vi "MiPS_turn_on_heater.vi"(6 "ISOBUS address":T4, 7 "switching_allowed":bool, 8 "error in":errorcluster, 9 "ref_in":T1, 10 "ref_slider":refnum<vi>, 11 "ref_big_msg":refnum<vi>) -> (0 "error out":errorcluster, 3 "ref_out":T1)   [LabVIEW 2019]
uses:
  Mercury iXX Modules/Public/Controls/ISOBus Address.ctl
  Mercury iXX Modules/Public/Controls/Mercury Reference.ctl
  Mercury iXX Modules/Public/Controls/Comms Transport Layer.ctl
  Mercury iXX Modules/Private/Controls/Query Dynamic Reference.ctl
  Mercury iXX Modules/Public/Libraries/Magnet/Controls/Switch Heater.ctl
  Mercury iXX Modules/Public/Libraries/Magnet/Signals/Set/Switch Heater No Check (Set).vi
  Mercury iXX Modules/Public/Libraries/Magnet.lvlib
  Mercury iXX Modules/Mercury iXX.lvlib
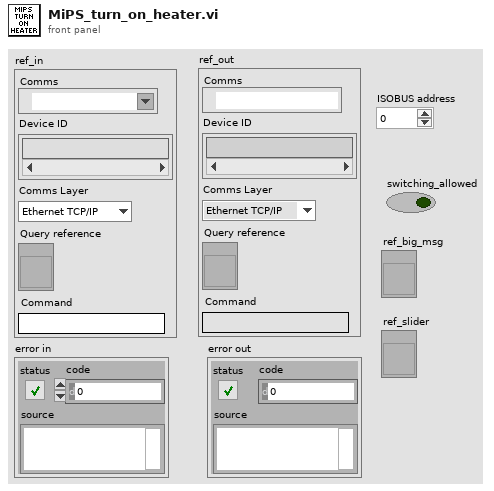
[diagram p1: front panel]
types:
  T1 = typedef "Mercury iXX.lvlib/Mercury Reference.ctl" = cluster{"Comms":refnum<visa-resource-name>, "Device ID":string[], "Comms Layer":T2, "Command":string, "Query reference":T3}
  T2 = typedef "Mercury iXX.lvlib/Comms Transport Layer.ctl" = enum16{"Ethernet TCP/IP", "USB", "ISOBus - RS-232", "GPIB"}
  T3 = typedef "Mercury iXX.lvlib/Query Dynamic Reference.ctl" = refnum<vi>
  T4 = typedef "Mercury iXX.lvlib/ISOBus Address.ctl" = i32
  T5 = typedef "Mercury iXX.lvlib/Magnet.lvlib/Switch Heater.ctl" = string
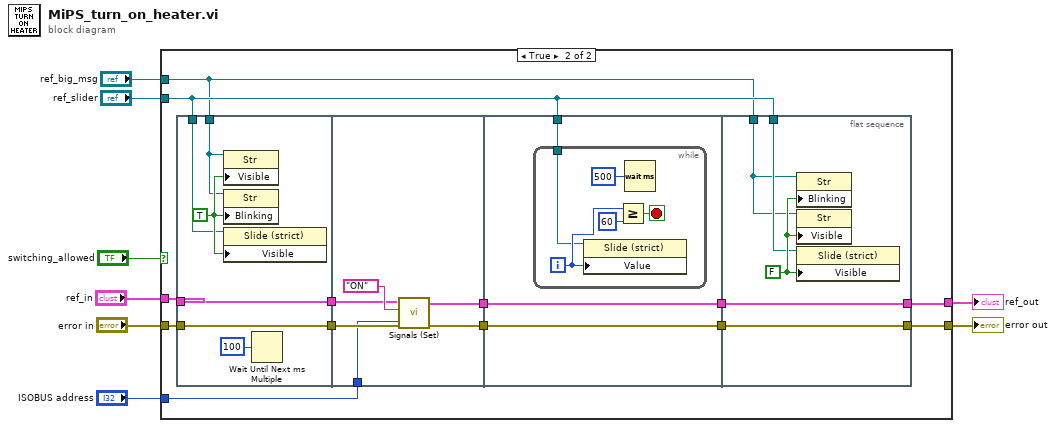
[diagram p0: block diagram]
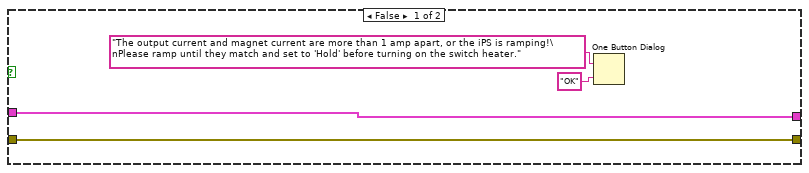
[diagram p2: hidden frame]
diagram:
  n1 = case shown="True" "switching_allowed" {
    tunnel: "ref_in" -> [w12 w20]
    tunnel: [w12 w25] -> w7
    tunnel: "error in" -> [w11 w18]
    tunnel: [w11 w24] -> w6
    tunnel: "ISOBUS address" -> [_ w17]
    tunnel: "ref_slider" -> [_ w14]
    tunnel: "ref_big_msg" -> [_ w13]
    frame False {
      n2 = One Button Dialog(message="The output current and magnet current are more than 1 amp apart, or the iPS is ramping!\nPlease ramp until they match and set to 'Hold' before turning on the switch heater.", button name ("OK")="OK") -> ()  [unwired: 1 out]
    }
    frame True {
      n3 = flat-sequence {
        tunnel: w20 -> [w30]
        tunnel: [w30] -> w21
        tunnel: [w29] -> w19
        tunnel: w18 -> [w29]
        tunnel: w13 -> [w27]
        tunnel: w14 -> [w26]
        tunnel: [w37] -> w16
        tunnel: [w36] -> w15
        tunnel: w21 -> [w34]
        tunnel: w19 -> [w33]
        tunnel: w17 -> [w32]
        tunnel: w16 -> [w40]
        tunnel: w15 -> [w39]
        tunnel: [w40] -> w23
        tunnel: [w39] -> w22
        tunnel: w14 -> [w38]
        tunnel: [w49] -> w24
        tunnel: [w50] -> w25
        tunnel: w23 -> [w50]
        tunnel: w22 -> [w49]
        tunnel: w14 -> [w47]
        tunnel: w13 -> [w46]
        frame #0 {
          w28 = TRUE ("Visible")
          n4 = property on="Property Node" class="Str"(reference=w27, "Visible"=w28) -> ()  [unwired: 1 in, 2 out]
          n5 = property on="Property Node" class="Str"(reference=w27, "Blinking"=w28) -> ()  [unwired: 1 in, 2 out]
          n6 = property on="Property Node" class="Slide (strict)"(reference=w26, "Visible"=w28) -> ()  [unwired: 1 in, 2 out]
          n7 = Wait Until Next ms Multiple(millisecond multiple=u32 100) -> ()  [unwired: 1 out]
        }
        frame #1 {
          n8 = call-poly "Signals (Set).vi"("ISOBUS address"=w32, "error in"=w33, "Set Switch Heater"=T5 "ON", "Mercury Reference In"=w34) -> ("error out"=w36:errorcluster, "Mercury Reference Out"=w37:T1)  [unwired: 4 in, 2 out]
        }
        frame #2 {
          n9 = while {
            tunnel: w38 -> [w41]
            i -> [w42]
            stop <- w44 stop-if-true
            n10 = property on="Property Node" class="Slide (strict)"(reference=w41, "Value"=w42) -> ()  [unwired: 1 in, 2 out]
            n11 = Greater Or Equal?(x=w42, y=60) -> (x >= y?=w44:bool)
            n12 = Wait (ms)(milliseconds to wait=u32 500) -> ()  [unwired: 1 out]
          }
        }
        frame #3 {
          w48 = FALSE ("Visible")
          n13 = property on="Property Node" class="Str"(reference=w46, "Blinking"=w48) -> ()  [unwired: 1 in, 2 out]
          n14 = property on="Property Node" class="Str"(reference=w46, "Visible"=w48) -> ()  [unwired: 1 in, 2 out]
          n15 = property on="Property Node" class="Slide (strict)"(reference=w47, "Visible"=w48) -> ()  [unwired: 1 in, 2 out]
        }
      }
    }
  }
  "ref_out" <- w7
  "error out" <- w6
